vi "slam_ortogonal_sem_odometria__(x,y).vi"() -> ()   [LabVIEW 2016]
uses:
  <vilib>/NXT/Subs/LVHSConnector.ctl
  <vilib>/NXT/LegoClasses/BrickReference/BrickReference.lvclass
  <vilib>/NXT/Block Support/NXT_OutputPort.ctl
  <vilib>/NXT/NXTIO Xnodes/NXTIONodeSubVIs/NXTStopMotors.vi
  <vilib>/NXT/NXTIO Xnodes/NXTIONodeSubVIs/NXTMoveMotors.vi
  <vilib>/NXT/Dual Mode Library/Waits/Wait_Num.vi
  <vilib>/NXT/NXTIO Xnodes/AddressXNode/NXTIOAddress.xnode
  <vilib>/NXT/NXTIO Xnodes/NXTIOXNode/NXTIO.xnode
panel:
  out "NXT/EV3 2":T1
  in  "NXT/EV3":T1
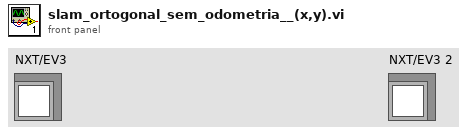
[diagram p1: front panel]
types:
  T1 = typedef "LVHSConnector.ctl" = refnum<class "BrickReference.lvclass">
  T2 = typedef "NXT_OutputPort.ctl" = u8
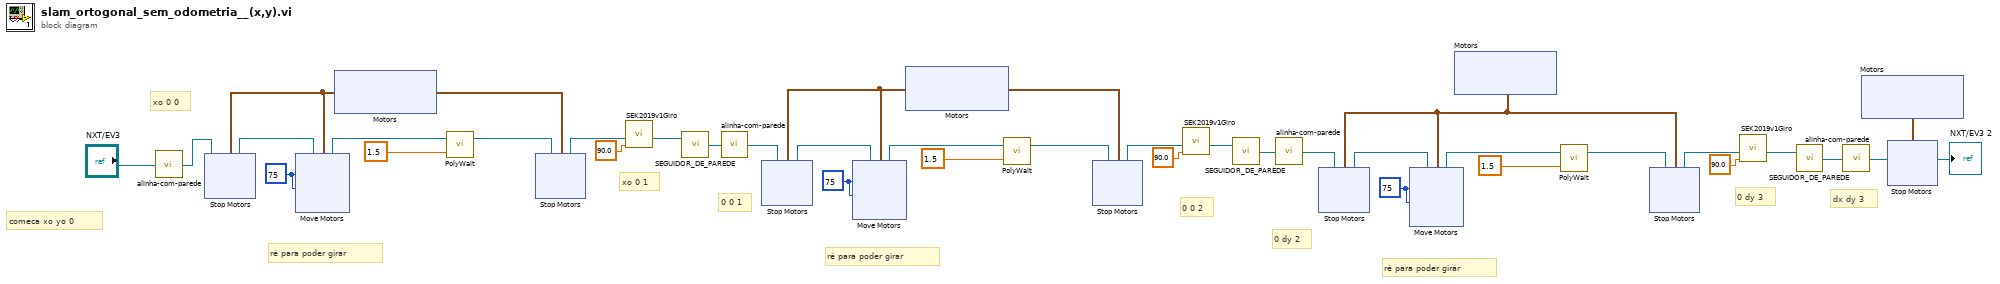
[diagram p0: block diagram]
diagram:
  w12 = i8 75 ("Power/Speed 1")
  w23 = i8 75 ("Power/Speed 1")
  w32 = i8 75 ("Power/Speed 1")
  # "dx dy 3"
  # "0 dy 3"
  # "ré para poder girar"
  # "0 dy 2"
  # "0 0 2"
  # "ré para poder girar"
  # "0 0 1"
  # "xo 0 1"
  # "ré para poder girar"
  # "xo 0 0"
  # "comeca xo yo 0"
  n1 = call "alinha-com-parede.vi"("NXT/EV3"="NXT/EV3") -> ("NXT/EV3 2"=w1:T1)  [unwired: 4 in]
  n2 = xnode "Motors"() -> ("Motor"=w28:cluster{"Port":T2, "Port":T2})
  n3 = xnode "Stop Motors"("Motors"=w28, "NXT/EV3"=w1) -> ("NXT/EV3"=w33:T1)
  n4 = xnode "Move Motors"("Power/Speed 2"=w32, "Power/Speed 1"=w32, "Motors"=w28, "NXT/EV3"=w33) -> ("NXT/EV3"=w34:T1)
  n5 = call-poly <vilib>:"PolyWait.vi"("Time (1 sec)"=sgl 1.5, "NXT/EV3"=w34) -> ("NXT/EV3"=w36:T1)  [unwired: 2 in]
  n6 = xnode "Stop Motors"("Motors"=w28, "NXT/EV3"=w36) -> ("NXT/EV3"=w31:T1)
  n7 = call "SEK2019v1Giro.vi"("ANGULO"=sgl 90.0, "NXT/EV3"=w31) -> ("NXT/EV3 2"=w29:T1)  [unwired: 9 in]
  n8 = call "SEGUIDOR_DE_PAREDE.vi"("NXT/EV3"=w29) -> ("NXT/EV3 2"=w27:T1)  [unwired: 1 in]
  n9 = call "alinha-com-parede.vi"("NXT/EV3"=w27) -> ("NXT/EV3 2"=w18:T1)  [unwired: 4 in]
  n10 = xnode "Motors"() -> ("Motor"=w26:cluster{"Port":T2, "Port":T2})
  n11 = xnode "Stop Motors"("Motors"=w26, "NXT/EV3"=w18) -> ("NXT/EV3"=w22:T1)
  n12 = xnode "Move Motors"("Power/Speed 2"=w23, "Power/Speed 1"=w23, "Motors"=w26, "NXT/EV3"=w22) -> ("NXT/EV3"=w21:T1)
  n13 = call-poly <vilib>:"PolyWait.vi"("Time (1 sec)"=sgl 1.5, "NXT/EV3"=w21) -> ("NXT/EV3"=w19:T1)  [unwired: 2 in]
  n14 = xnode "Stop Motors"("Motors"=w26, "NXT/EV3"=w19) -> ("NXT/EV3"=w24:T1)
  n15 = call "SEK2019v1Giro.vi"("ANGULO"=sgl 90.0, "NXT/EV3"=w24) -> ("NXT/EV3 2"=w8:T1)  [unwired: 9 in]
  n16 = call "SEGUIDOR_DE_PAREDE.vi"("NXT/EV3"=w8) -> ("NXT/EV3 2"=w9:T1)  [unwired: 1 in]
  n17 = call "alinha-com-parede.vi"("NXT/EV3"=w9) -> ("NXT/EV3 2"=w17:T1)  [unwired: 4 in]
  n18 = xnode "Motors"() -> ("Motor"=w2:cluster{"Port":T2, "Port":T2})
  n19 = xnode "Stop Motors"("Motors"=w2, "NXT/EV3"=w17) -> ("NXT/EV3"=w13:T1)
  n20 = xnode "Move Motors"("Power/Speed 2"=w12, "Power/Speed 1"=w12, "Motors"=w2, "NXT/EV3"=w13) -> ("NXT/EV3"=w14:T1)
  n21 = call-poly <vilib>:"PolyWait.vi"("Time (1 sec)"=sgl 1.5, "NXT/EV3"=w14) -> ("NXT/EV3"=w16:T1)  [unwired: 2 in]
  n22 = xnode "Stop Motors"("Motors"=w2, "NXT/EV3"=w16) -> ("NXT/EV3"=w11:T1)
  n23 = call "SEK2019v1Giro.vi"("ANGULO"=sgl 90.0, "NXT/EV3"=w11) -> ("NXT/EV3 2"=w4:T1)  [unwired: 9 in]
  n24 = call "SEGUIDOR_DE_PAREDE.vi"("NXT/EV3"=w4) -> ("NXT/EV3 2"=w7:T1)  [unwired: 1 in]
  n25 = call "alinha-com-parede.vi"("NXT/EV3"=w7) -> ("NXT/EV3 2"=w5:T1)  [unwired: 4 in]
  n26 = xnode "Motors"() -> ("Motor"=w6:cluster{"Port":T2, "Port":T2})
  n27 = xnode "Stop Motors"("Motors"=w6, "NXT/EV3"=w5) -> ("NXT/EV3"=→"NXT/EV3 2":T1)
